vi "BRig_dataExp_CueSwitch_First.vi"() -> (2 "output_CueSwitch_First":i32)   [LabVIEW 2014]
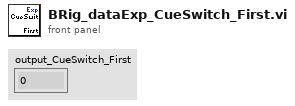
[diagram p1: front panel]
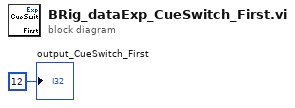
[diagram p0: block diagram]
diagram:
  "output_CueSwitch_First" <- 12 ("output_iBlock")
